vi "ClosestPoint.vi"(10 "Robot":cluster{"x":dbl, "y":dbl}, 11 "Path":cluster{"x":dbl, "y":dbl}[](array[cluster])) -> (1 "Distance":dbl, 2 "Index":i32, 3 "Point":cluster{"x":dbl, "y":dbl})   [LabVIEW 2016]
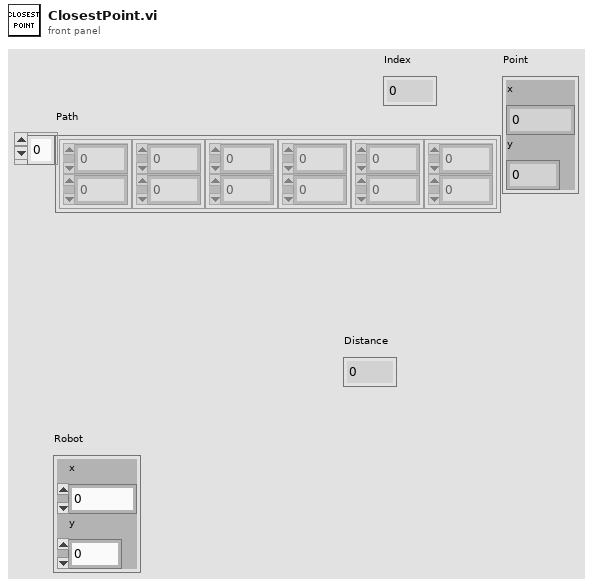
[diagram p1: front panel]
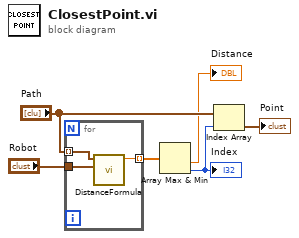
[diagram p0: block diagram]
diagram:
  n1 = for {
    tunnel: "Robot" -> [w9]
    tunnel: "Path" -> [w8] mode=indexing
    tunnel: [w7] -> w5 mode=indexing
    n2 = call "DistanceFormula.vi"("Point 2"=w9, "Point 1"=w8) -> ("Distance"=w7:dbl)  [unwired: 9 in]
  }
  n3 = Array Max & Min(array=w5) -> (min value=→"Distance":dbl, min index (indices)=w2:i32)  [unwired: 2 out]
  "Index" <- w2
  n4 = Index Array(array="Path", index=w2) -> (element=→"Point":cluster{"x":dbl, "y":dbl})
